vi "overheat control.vi"() -> ()   [LabVIEW 2010]
panel:
  out "Overheat !!":bool
  in  "Over heat \nTemperature":dbl
  in  "Overheat protection":bool
  in  "Control Gas flow ?":bool=TRUE
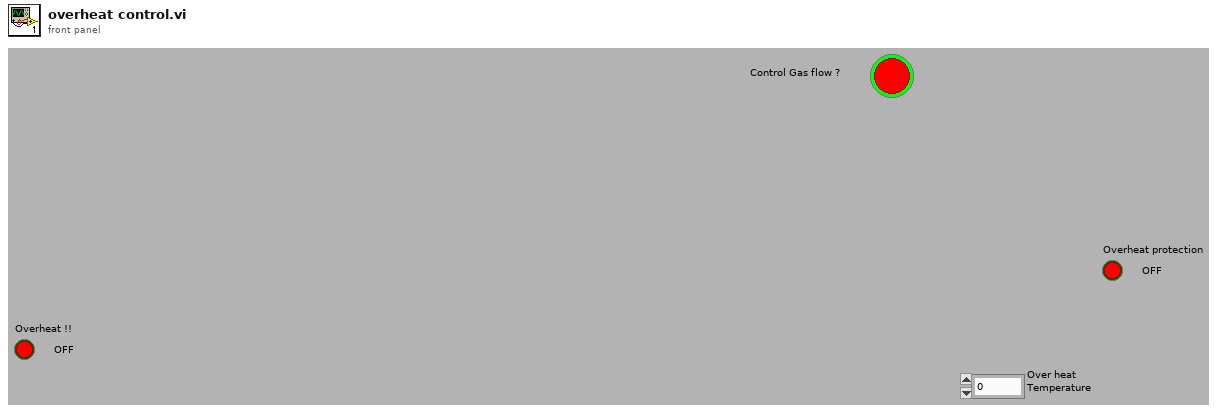
[diagram p1: front panel]
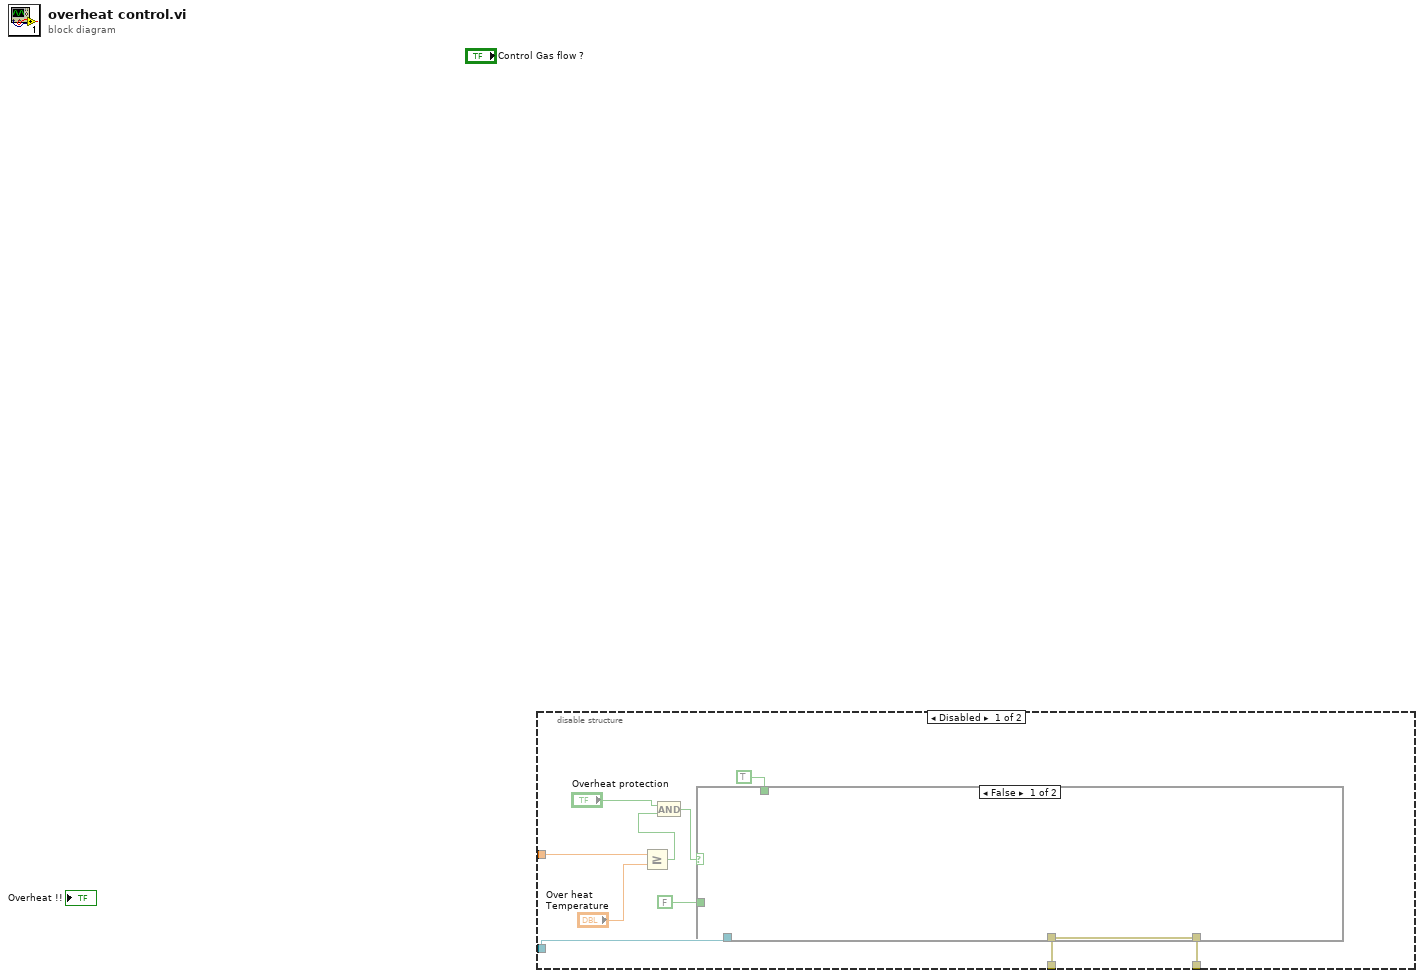
[diagram p0: block diagram]
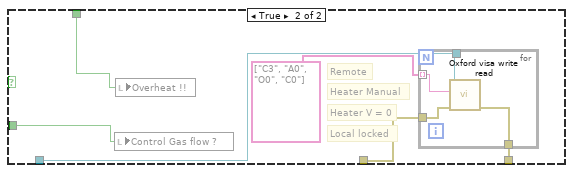
[diagram p2: hidden frame]
diagram:
  n1 = disable-structure shown="Disabled" {
    disable-tunnel: _ -> [w4 _]
    disable-tunnel: _ -> [w3 _]
    disable-tunnel: _ -> [w2 w22]
    disable-tunnel: [w1 w22] -> _
    frame Disabled {
      n2 = Greater Or Equal?(x=w4, y="Over heat \nTemperature") -> (x >= y?=w8:bool)
      n3 = And(x="Overheat protection", y=w8) -> (x .and. y?=w7:bool)
      n4 = case shown="False" w7 {
        tunnel: w3 -> [_ w17]
        tunnel: FALSE ("Control Gas flow ?") -> [_ w14]
        tunnel: TRUE ("Boolean") -> [_ w15]
        tunnel: w2 -> [w11 w13]
        tunnel: [w11 w12] -> w1
        frame False {
        }
        frame True {
          # "Local locked"
          # "Heater V = 0"
          # "Heater Manual"
          # "Remote"
          n5 = local write "Control Gas flow ?"(w14) -> ()
          n6 = local write "Overheat !!"(w15) -> ()
          n7 = for {
            tunnel: w17 -> [w21]
            tunnel: string[] ["C3", "A0", "O0", "C0"] -> [w20] mode=indexing
            tunnel: w13 -> [w19]
            tunnel: [w18] -> w12
            n8 = call "Oxford visa write read.vi"("error in (no error)"=w19, "write buffer"=w20, "VISA resource name"=w21) -> ("error out"=w18:errorcluster)  [unwired: 6 in, 2 out]
          }
        }
      }
    }
    frame Enabled {
    }
  }
